vi "删除一条记录.vi"(9 "ID":i32) -> ()   [LabVIEW 2010]
panel:
  in  "error in (no error) 2":errorcluster caption="错误输入（无错误）"
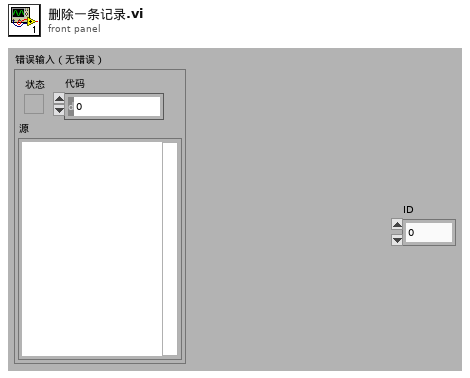
[diagram p1: front panel]
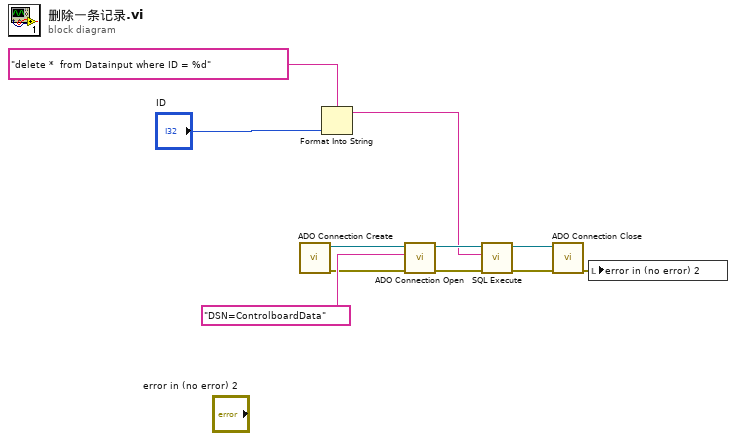
[diagram p0: block diagram]
diagram:
  n1 = call "ADO Connection Create.vi"() -> ("error out"=w5:errorcluster, "ADODB._Connection Out"=w4:refnum<k7>)  [unwired: 10 in]
  n2 = Format Into String(format string="delete *  from Datainput where ID = %d", "ID") -> (resulting string=w2:string)  [unwired: 2 in, 1 out]
  n3 = call "ADO Connection Open.vi"("error in (no error)"=w5, "ConnectionString"="DSN=ControlboardData", "ADODB._Connection In"=w4) -> ("error out"=w8:errorcluster, "ADODB._Connection Out"=w11:refnum<k7>)  [unwired: 7 in]
  n4 = call "SQL Execute.vi"("error in (no error)"=w8, "Command Text"=w2, "ADODB._Connection In"=w11) -> ("error out"=w7:errorcluster, "ADODB._Connection Out"=w10:refnum<k7>)  [unwired: 5 in, 2 out]
  n5 = call "ADO Connection Close.vi"("error in (no error)"=w7, "ADODB._Connection In"=w10) -> ("error out"=w6:errorcluster)  [unwired: 8 in, 1 out]
  n6 = local write "error in (no error) 2"(w6) -> ()
